vi "test.vi"() -> ()   [LabVIEW 2018]
uses:
  <vilib>/Utility/inputDevices.llb/joystickAcquire.vi
panel:
  out "axis info":T1
  out "Wheel Speeds [-1..1]":dbl[](array[numeric])
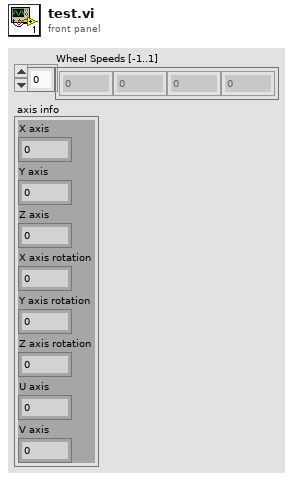
[diagram p1: front panel]
types:
  T1 = cluster{"X axis":i32, "Y axis":i32, "Z axis":i32, "X axis rotation":i32, "Y axis rotation":i32, "Z axis rotation":i32, "U axis":i32, "V axis":i32}
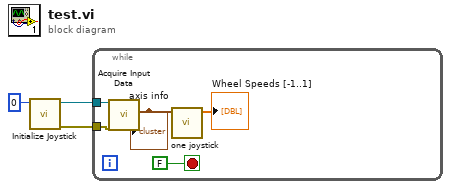
[diagram p0: block diagram]
diagram:
  n1 = call <vilib>:"Initialize Joystick.vi"("device index"=0) -> ("error out"=w2:errorcluster, "device ID"=w3:refnum<k1>)  [unwired: 9 in]
  n2 = while {
    tunnel: w3 -> [w7]
    tunnel: w2 -> [w6]
    stop <- FALSE stop-if-true
    n3 = call-poly <vilib>:"Acquire Input Data.vi"("device ID"=w7, "error in (no error)"=w6) -> ("axis info"=w5:T1)  [unwired: 13 in, 4 out]
    "axis info" <- w5
    n4 = call <vilib>:"one joystick.vi"("axis info"=w5) -> ("Wheel Speeds [-1..1]"=→"Wheel Speeds [-1..1]":dbl[])  [unwired: 10 in]
  }
